vi "BeeperData_Validation.vi"(0 "offset":dbl=131.6, 1 "path":path=path "C:/mtp/Site_Ne_sch/Projects/AVALANCHE/CUSTOM/BeeperData/14251010502229-Beeper_9_50_56.wav", 4 "Upper Cut-Off":dbl=15000.0, 5 "Lower Cut-Off":dbl=2000.0) -> (10 "N Harmonics":i32=1, 12 "Harmonic Array":T1(array[cluster])=[{"detected frequency"=2960.3023758852505, "detected amplitude"=100.09262427578935, "detected phase (deg)"=21.541772749437428}], 13 "error out":errorcluster, 14 "PASS/FAIL 4":bool=TRUE caption="PASS/FAIL", 15 "fundamental frequency":dbl=2934.715709878751 format="%.2p", 16 "fundamental amplitude":dbl=0.025259592284939396, 17 "fundamental dB output":dbl=99.6485267265794, 18 "THD":dbl=9.755635404697069 format="%.2p")   [LabVIEW 2014]
uses:
  <vilib>/express/express analysis/Spectral/Block/exnSpectralBlock spectral measurements peak poly.vi
  <vilib>/express/express analysis/Spectral/Block/exnSpectralBlock spectral measurements peak WFM.vi
  <vilib>/measure/matone.llb/Extract Multiple Tone Information 1 Chan.vi
  <vilib>/measure/matone.llb/Harmonic Distortion Analyzer 1 Chan.vi
  <vilib>/express/express analysis/Spectral/XNode/ExpressSpectralMeasurementsBlockNode.xnode
  <vilib>/measure/NI_MAPro.lvlib
panel:
  out "max index(es)":i32=1
  out "components level":dbl[](array[numeric])=[-2.401233861026392e-07, 0.025259592284939396, 0.002224247422714069, 0.00081423605464637, 0.000593690234948729, 0.00033120473717450035, 5.1228130884612615e-06, 4.283185131983852e-09, 2.0407182090206694e-10] format="%.2p"
  out "Beeper Time Domain AC":waveform(dbl)(graph)={"t0"=timestamp(0.0010416666666666667 s since 1904-01-01), "dt"=2.0833333333333333e-05, "Y"=array[455 elements], "attributes"=variant("NI_ChannelName"=variant(string "Filtered (Extracted)"), "NI_ExpIsRelativeTime"=variant(bool TRUE), "NI_ExpStartTimeStamp"=variant(timestamp timestamp(3493299977.1484375 s since 1904-01-01)), "NI_ExpTimeStamp"=variant(timestamp timestamp(3493299977.1494794 s since 1904-01-01)), "NI_ExpXDimension"=variant(string "t"), "NI_OriginalChannelName"=variant(string "Filtered"))}
  out "FFT Mask":dynamicdata(graph)=[{"t0"=timestamp(-68399 s since 1904-01-01), "dt"=105.49450549450549, "Y"=array[228 elements]}, {"t0"=timestamp(-68399 s since 1904-01-01), "dt"=105.49450549450549, "Y"=[nan, nan, nan, nan, nan, nan, nan, nan, nan, nan, nan, nan, nan, nan, nan, nan, nan, nan, nan, nan, nan, nan, nan, nan, nan, nan, nan, nan, nan, nan, nan, nan, nan, nan, nan, nan, nan, nan, nan, nan, nan, nan, nan, nan, nan, nan, nan, nan, nan, nan, nan, nan, nan, nan, nan, nan, nan, nan, nan, nan, nan, nan, nan, nan, nan, nan, nan, nan, nan, nan, nan, nan, nan, nan, nan, nan, nan, nan, nan, nan, nan, nan, nan, nan, nan, nan, nan, nan, nan, nan, nan, nan, nan, nan, nan, nan, nan, nan, nan, nan, nan, nan, nan, nan, nan, nan, nan, nan, nan, nan, nan, nan, nan, nan, nan, nan, nan, nan, nan, nan, nan, nan, nan, nan, nan, nan, nan, nan, nan, nan, nan, nan, nan, nan, nan, nan, nan, nan, nan, nan, nan, nan, nan, nan, nan, nan, nan, nan, nan, nan, nan, nan, nan, nan, nan, nan, nan, nan, nan, nan, nan, nan, nan, nan, nan, nan, nan, nan, nan, nan, nan, nan, nan, nan, nan, nan, nan, nan, nan, nan, nan, nan, nan, nan, nan, nan, nan, nan, nan, nan, nan, nan, nan, nan, nan, nan, nan, nan, nan, nan, nan, nan, nan, nan, nan, nan, nan, nan, nan, nan, nan, nan, nan, nan, nan, nan, nan, nan, nan, nan, nan, nan, nan, nan, nan, nan, nan, nan], "attributes"=variant("NI_ChannelName"=variant(string "Failures"))}, {"t0"=timestamp(-68399 s since 1904-01-01), "dt"=105.49450549450549, "Y"=[3.0, 3.0, 3.0, 3.0, 3.0, 2.9700353311878396, 2.916806756284134, 2.8635781813804284, 2.8103496064767235, 2.7571210315730177, 2.7038924566693128, 2.650663881765607, 2.5974353068619016, 2.5442067319581962, 2.490978157054491, 2.4377495821507855, 2.38452100724708, 2.331292432343375, 2.2780638574396694, 2.224835282535964, 2.1716067076322587, 2.118378132728553, 2.065149557824848, 2.011920982921142, 70.0, 70.0, 70.0, 70.0, 70.0, 70.0, 70.0, 70.0, 70.0, 70.0, 2.0, 2.0, 2.0, 2.0, 2.0, 2.0, 2.0, 2.0, 2.0, 2.0, 2.0, 2.0, 2.0, 2.0, 2.0, 2.0, 2.0, 2.0, 36.285714285714114, 50.0, 50.0, 50.0, 50.0, 50.0, 50.0, 50.0, 50.0, 50.0, 10.967032967033415, 2.0, 2.0, 2.0, 2.0, 2.0, 2.0, 2.0, 2.0, 2.0, 2.0, 2.0, 2.0, 2.0, 2.0, 2.0, 2.0, 2.0, 2.0, 20.0, 20.0, 20.0, 20.0, 20.0, 20.0, 20.0, 20.0, 20.0, 20.0, 2.0, 2.0, 2.0, 2.0, 2.0, 2.0, 2.0, 2.0, 2.0, 2.0, 2.0, 2.0, 2.0, 2.0, 2.0, 2.0, 2.0, 2.0, 2.0, 2.0, 2.0, 2.0, 2.0, 2.0, 2.0, 2.0, 2.0, 2.0, 2.0, 2.0, 2.0, 2.0, 2.0, 2.0, 2.0, 2.0, 2.0, 2.0, 2.0, 2.0, 2.0, 2.0, 2.0, 2.0, 2.0, 2.0, 2.0, 2.0, 2.0, 2.0, 2.0, 2.0, 2.0, 2.0, 2.0, 2.0, 2.0, 2.0, 2.0, 2.0, 2.0, 2.0, 2.0, 2.0, 2.0, 2.0, 2.0, 2.0, 2.0, 2.0, 2.0, 2.0, 2.0, 2.0, 2.0, 2.0, 2.0, 2.0, 2.0, 2.0, 2.0, 2.0, 2.0, 2.0, 2.0, 2.0, 2.0, 2.0, 2.0, 2.0, 2.0, 2.0, 2.0, 2.0, 2.0, 2.0, 2.0, 2.0, 2.0, 2.0, 2.0, 2.0, 2.0, 2.0, 2.0, 2.0, 2.0, 2.0, 2.0, 2.0, 2.0, 2.0, 2.0, 2.0, 2.0, 2.0, 2.0, 2.0, 2.0, 2.0, 2.0, 2.0, 2.0, 2.0, 2.0, 2.0, 2.0, 2.0, 2.0, 2.0, 2.0, 2.0, 2.0, 2.0, 2.0, 2.0, 2.0], "attributes"=variant("NI_ChannelName"=variant(string "Upper Limit"))}, {"t0"=timestamp(-68399 s since 1904-01-01), "dt"=105.49450549450549, "Y"=[0.0, 0.0, 0.0, 0.0, 0.0, 0.0, 0.0, 0.0, 0.0, 0.0, 0.0, 0.0, 0.0, 0.0, 0.0, 0.0, 0.0, 0.0, 0.0, 0.0, 0.0, 0.0, 0.0, 0.0, 0.0, 0.0, 0.0, 0.0, 0.0, 0.0, 0.0, 0.0, 0.0, 0.0, 0.0, 0.0, 0.0, 0.0, 0.0, 0.0, 0.0, 0.0, 0.0, 0.0, 0.0, 0.0, 0.0, 0.0, 0.0, 0.0, 0.0, 0.0, 0.0, 0.0, 0.0, 0.0, 0.0, 0.0, 0.0, 0.0, 0.0, 0.0, 0.0, 0.0, 0.0, 0.0, 0.0, 0.0, 0.0, 0.0, 0.0, 0.0, 0.0, 0.0, 0.0, 0.0, 0.0, 0.0, 0.0, 0.0, 0.0, 0.0, 0.0, 0.0, 0.0, 0.0, 0.0, 0.0, 0.0, 0.0, 0.0, 0.0, 0.0, 0.0, 0.0, 0.0, 0.0, 0.0, 0.0, 0.0, 0.0, 0.0, 0.0, 0.0, 0.0, 0.0, 0.0, 0.0, 0.0, 0.0, 0.0, 0.0, 0.0, 0.0, 0.0, 0.0, 0.0, 0.0, 0.0, 0.0, 0.0, 0.0, 0.0, 0.0, 0.0, 0.0, 0.0, 0.0, 0.0, 0.0, 0.0, 0.0, 0.0, 0.0, 0.0, 0.0, 0.0, 0.0, 0.0, 0.0, 0.0, 0.0, 0.0, 0.0, 0.0, 0.0, 0.0, 0.0, 0.0, 0.0, 0.0, 0.0, 0.0, 0.0, 0.0, 0.0, 0.0, 0.0, 0.0, 0.0, 0.0, 0.0, 0.0, 0.0, 0.0, 0.0, 0.0, 0.0, 0.0, 0.0, 0.0, 0.0, 0.0, 0.0, 0.0, 0.0, 0.0, 0.0, 0.0, 0.0, 0.0, 0.0, 0.0, 0.0, 0.0, 0.0, 0.0, 0.0, 0.0, 0.0, 0.0, 0.0, 0.0, 0.0, 0.0, 0.0, 0.0, 0.0, 0.0, 0.0, 0.0, 0.0, 0.0, 0.0, 0.0, 0.0, 0.0, 0.0, 0.0, 0.0, 0.0, 0.0, 0.0, 0.0, 0.0, 0.0, 0.0, 0.0, 0.0, 0.0, 0.0, 0.0, 0.0, 0.0, 0.0, 0.0, 0.0, 0.0], "attributes"=variant("NI_ChannelName"=variant(string "Lower Limit"))}]
  out "Beeper Time Domain DC":waveform(dbl)(graph)={"t0"=timestamp(0 s since 1904-01-01), "dt"=2.0833333333333333e-05, "Y"=array[505 elements]}
  out "FFT Peak":cluster{"f0":dbl, "df":dbl, "magnitude":dbl[]}(graph)={"f0"=0.0, "df"=105.49450549450549, "magnitude"=[1.6018368008824488e-07, 2.739165277402443e-07, 3.985203981044255e-07, 5.917708316720877e-07, 8.748145112128303e-07, 1.3010814410825855e-06, 2.0802062107375216e-06, 2.790134744566662e-06, 5.753123783912797e-06, 1.4763146182645159e-05, 4.238164606283932e-06, 0.00012007636572453463, 0.00045236073044393853, 0.002934004193699415, 0.00618501386299634, 0.0064880498159982855, 0.004538550933487086, 0.005199055511354578, 0.006129575152514394, 0.006903653173956658, 0.00730576670286189, 0.007351995343235854, 0.007013327451583518, 0.006509554866980719, 0.006228470853974282, 0.0059152113548739315, 0.005498597813254141, 0.016062761736819666, 0.02472840707265435, 0.014786365312579881, 0.00239181992405032, 0.0021946637725328354, 0.0016716329640382012, 0.0022855801600055793, 0.0020901873459184686, 0.0017113901006194504, 0.001620746494749405, 0.0015562218927555732, 0.0013615690730541976, 0.0012180416934189037, 0.001119963237415986, 0.0012235355092325316, 0.004180665312898901, 0.0043012327175093144, 0.001612474254557478, 0.0014550970818332164, 0.002184396771928845, 0.0015683282438508053, 0.0015113981640458374, 0.0018553299437078332, 0.001432021634658514, 0.0012923059165754112, 0.0011823857826419426, 0.0010576757189758696, 0.0011219595762485385, 0.0004573132325211268, 0.0015561090460205571, 0.0021222291843564127, 0.0013223324797204017, 0.0011297547810841938, 0.0009469486200130573, 0.001072221032431467, 0.0010140248379210456, 0.0009535198860453821, 0.0009713855535785712, 0.0009733887927467716, 0.0009231871530565895, 0.0008862720858397985, 0.0008697663729143937, 0.0008808024231401676, 0.0008311296857765208, 0.0007683276179268573, 0.0007961849804113151, 0.0007876581727953233, 0.0007888359132087923, 0.000769776362911128, 0.0007402871142191691, 0.0007523865145557025, 0.0007307766379216526, 0.0007212053921743106, 0.0007221095514331676, 0.0007113072058043807, 0.0007071121006542068, 0.0006742963491071851, 0.0006427924843893649, 0.0006870497263242136, 0.0006749536371613217, 0.0006613102492586514, 0.0006489994908067029, 0.0006293390742419889, 0.0006363895989919498, 0.0006288592489611338, 0.0006141636133007902, 0.0005998170467609775, 0.000606898767172136, 0.0006100954906706817, 0.0005950655468311286, 0.0005687631384143958, 0.000645402197941972, 0.0006093938618635512, 0.0005440439587081989, 0.0005491501408034803, 0.0005471993333521795, 0.000555731215915673, 0.0005448049609387473, 0.0005268014591564282, 0.0005276165035064028, 0.0005193301431807729, 0.0005176891895592861, 0.0005071285001398295, 0.0005128221736897446, 0.0004946929370202132, 0.00020655127828846196, 0.0005833042883385348, 0.0005986223100015384, 0.000514062759255501, 0.0005162656836314005, 0.0004947426900875093, 0.0004900740942022137, 0.0005128959777501746, 0.0004962426346107286, 0.0004480936091845419, 0.0004677545173529926, 0.0004916103843928828, 0.00046833095017899206, 0.0004561521011779545, 0.0005351975121194499, 0.00048074459952987807, 0.0004019354125465926, 0.0004328421538882473, 0.0004177256245699992, 0.000401433108737401, 0.00040727619876232895, 0.00039014492249631315, 0.00037122537926854093, 0.0003572568717356956, 0.0003347011841836008, 0.000317645831002189, 0.00029499272337436887, 0.0002655709639012852, 0.0002456444610692289, 0.0002979351613877896, 0.0002488337977494649, 0.00021442893771735202, 0.00019253195485906686, 0.00016871746475827094, 0.00014708573773234747, 0.0001316727205698442, 0.00011475346989928615, 9.999567957957976e-05, 8.355183515284517e-05, 7.455418882715166e-05, 6.299284392853712e-05, 5.120665746323067e-05, 4.774908197114614e-05, 4.391330974930402e-05, 3.181851168252048e-05, 2.7269674200429926e-05, 2.221941603966412e-05, 1.8772239623046817e-05, 1.525105733418944e-05, 1.268089996340142e-05, 1.0235236333480283e-05, 8.551419418824312e-06, 6.9648649934696785e-06, 5.701748469266331e-06, 4.6962748957860825e-06, 3.922975065968365e-06, 3.067600106921259e-06, 2.530168944911267e-06, 2.068764944567118e-06, 1.666524485415195e-06, 1.3596624429221118e-06, 1.0836402074972496e-06, 8.989168769003971e-07, 7.197165570656004e-07, 5.481961280152284e-07, 4.472978961163214e-07, 3.637035768405892e-07, 2.787960899093122e-07, 2.1910979507048683e-07, 1.7296865493676617e-07, 1.3617842183839526e-07, 1.0468236401971942e-07, 8.287618712431156e-08, 6.33389189173673e-08, 4.785647426903807e-08, 3.652941249268399e-08, 3.04849648281208e-08, 2.265482254064642e-08, 1.6678952098245288e-08, 1.1962707544068855e-08, 9.019654193848143e-09, 7.257736329668531e-09, 4.61540575313361e-09, 3.0634685329644013e-09, 3.0153156852308272e-09, 1.981309720589669e-09, 7.567519387012121e-10, 1.1198464971128534e-09, 1.0079345420920498e-09, 8.701582864538078e-10, 1.3927584173258147e-09, 1.0723596774364627e-09, 3.4216758540295366e-10, 4.429352546738541e-10, 4.4336447100413793e-10, 3.6791998346199263e-10, 3.684405363850955e-10, 3.7838754731252655e-10, 3.5788638668105033e-10, 3.4703595026039633e-10, 3.4356000066506645e-10, 3.3494943254810104e-10, 3.269648763852098e-10, 3.208964950838077e-10, 3.147313728415835e-10, 3.0891418933647756e-10, 3.0373615893461565e-10, 2.9901971109520886e-10, 2.9478708873471836e-10, 2.9106814410454076e-10, 2.878628402777732e-10, 2.851786402689724e-10, 2.8302272856028055e-10, 2.814006053361294e-10, 2.803166559304008e-10, 2.797739135846308e-10]}
  # "Trigger at 0.8"
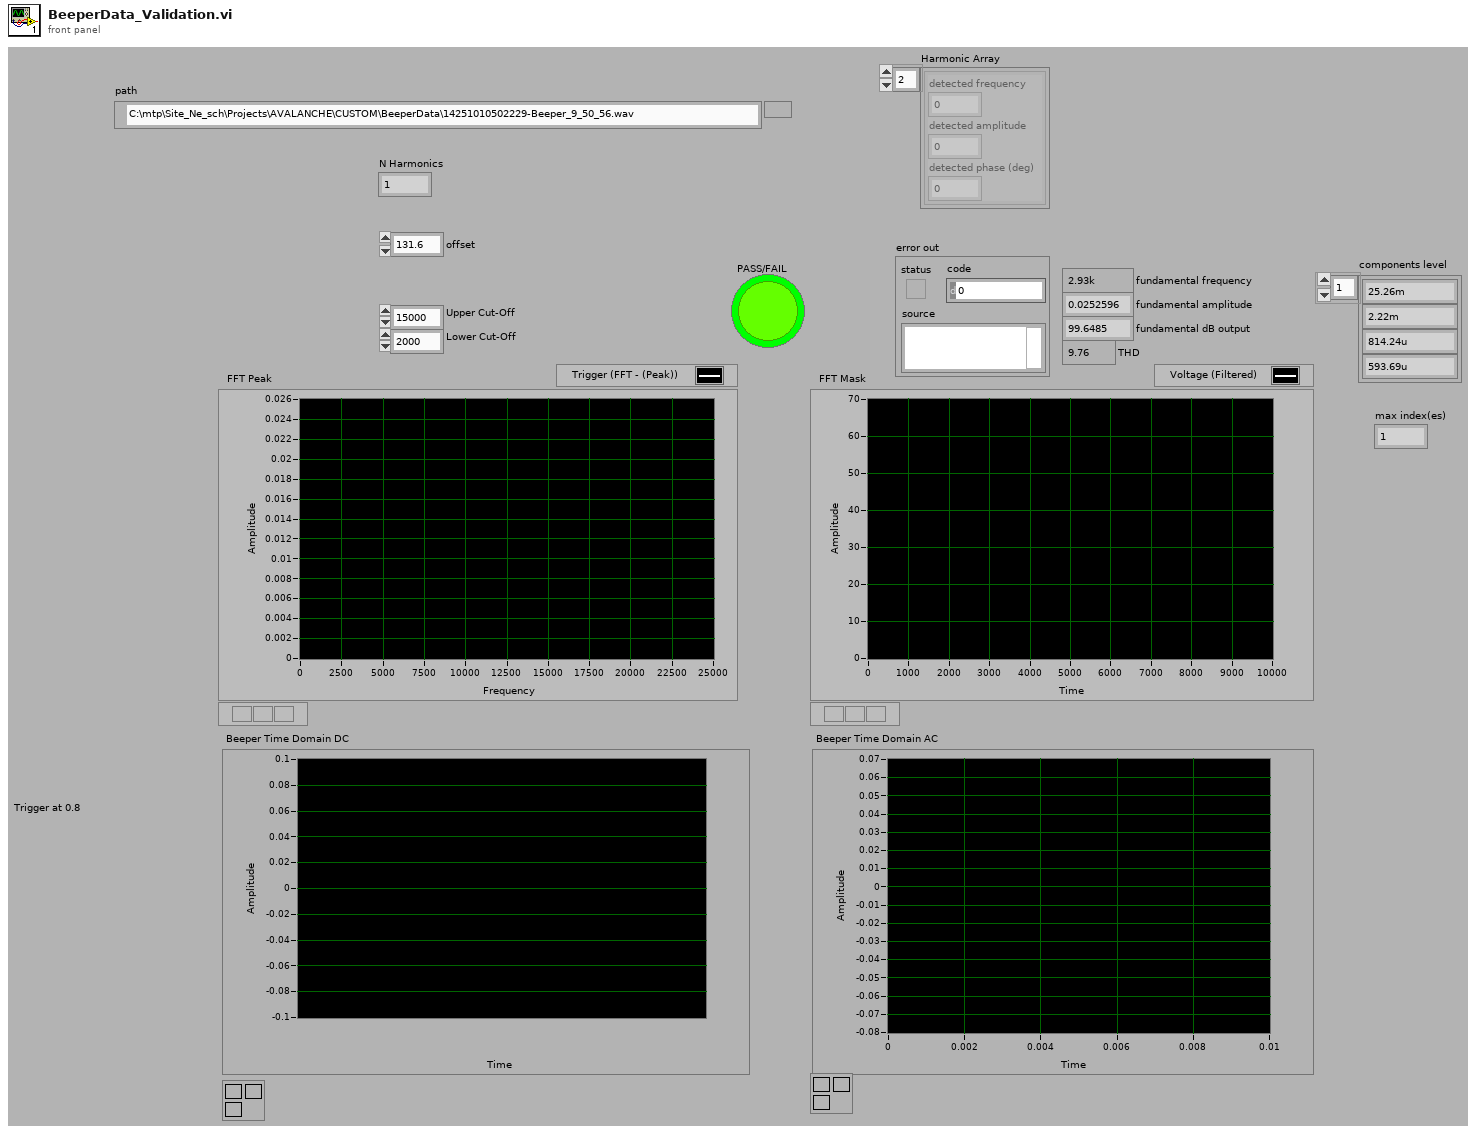
[diagram p1: front panel]
types:
  T1 = cluster{"detected frequency":dbl, "detected amplitude":dbl, "detected phase (deg)":dbl}[]
  T2 = cluster{"averaging mode":u16, "weighting mode":u16, "number of averages":u32}
  T3 = cluster{"dB On (F)":bool, "unwrap phase (F)":bool, "convert to degree (F)":bool}
  T4 = cluster{"approx freq. (optional)":dbl, "search (+/- % of Fsampl.)":dbl}
  T5 = enum32{"none", "input signal", "detected signal", "residual signal"}
  T6 = enum16{"none", "input signal", "fundamental signal", "residual signal", "harmonics only", "noise and spurs"}
  T7 = cluster{"detected frequency":dbl, "detected amplitude":dbl, "detected phase (deg)":dbl}
  T8 = cluster{"detected frequency":dbl, dbl, "detected phase (deg)":dbl}
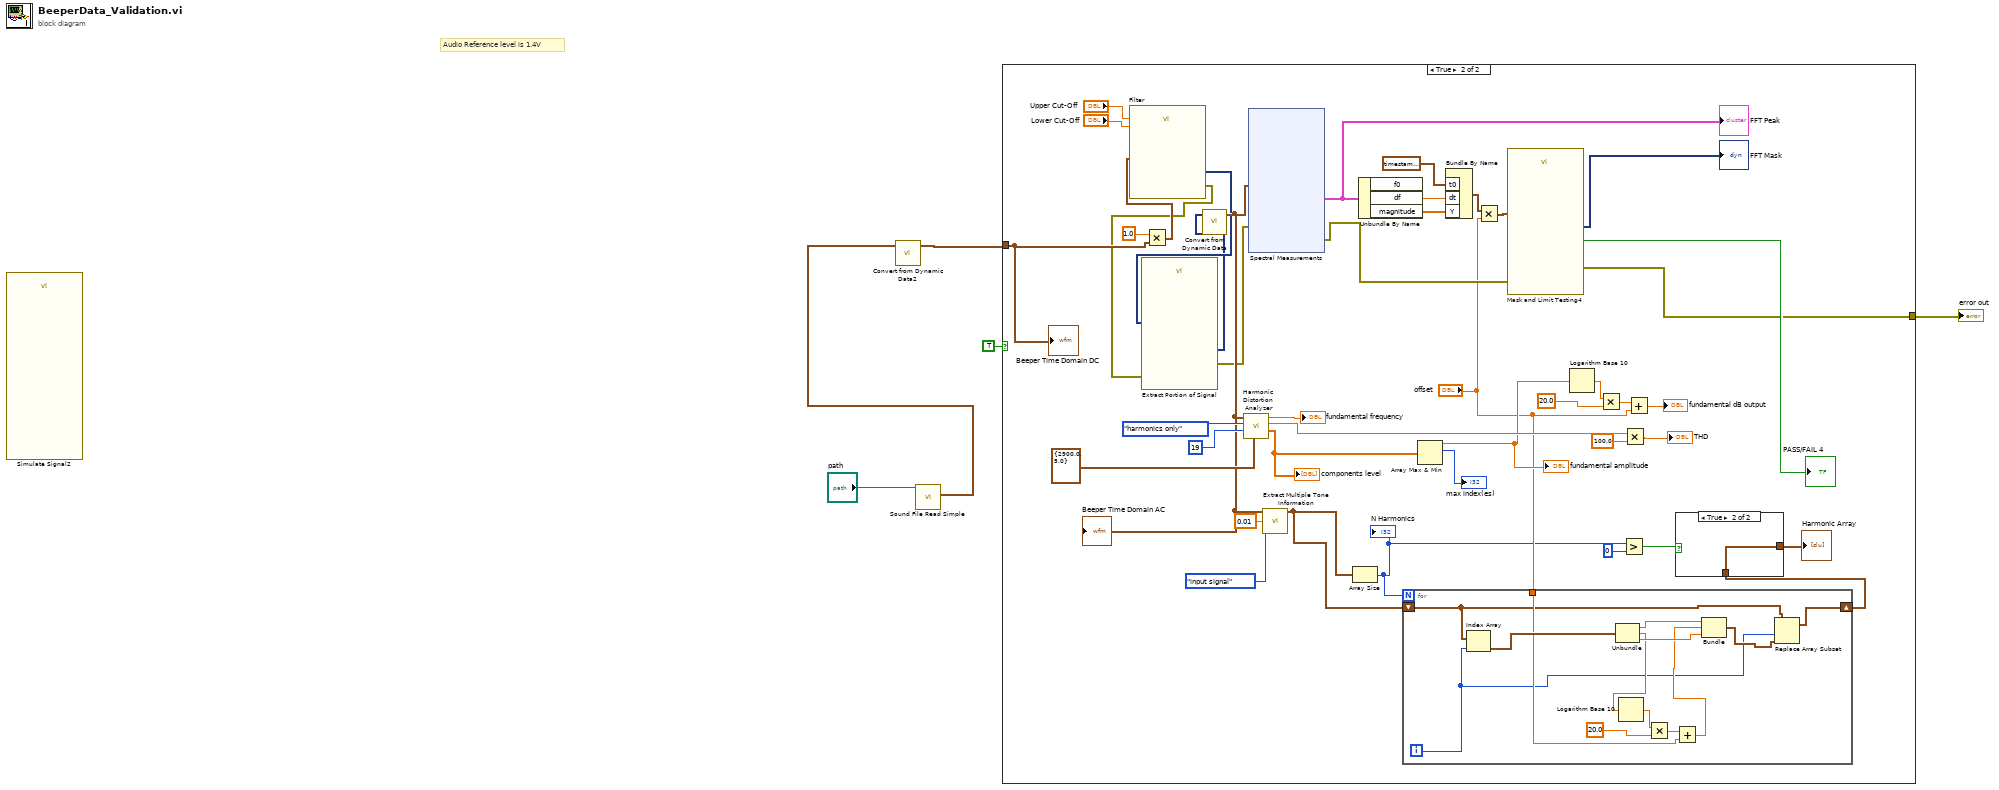
[diagram p0: block diagram]
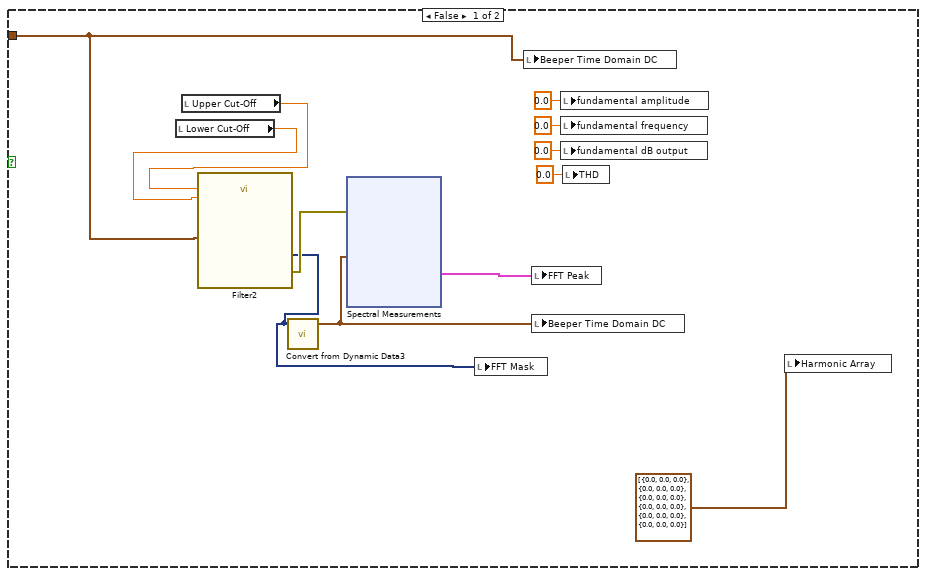
[diagram p2: hidden frame]
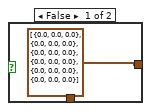
[diagram p3: hidden frame]
diagram:
  # "Audio Reference level is 1.4V"
  n1 = call "Simulate Signal2"() -> ()  [unwired: 14 in, 2 out]
  n2 = call <vilib>:"Sound File Read Simple.vi"("path"="path") -> ("data"=w2:waveform(dbl)[])  [unwired: 7 in, 3 out]
  n3 = call "Convert from Dynamic Data2"("Dynamic Data Type"=w2) -> ("Waveform"=w3:waveform(dbl))  [unwired: 3 in]
  n4 = case shown="True" TRUE {
    tunnel: w3 -> [w11 w47]
    tunnel: [_ w68] -> w5
    frame False {
      n5 = local read "Lower Cut-Off"() -> (w8:dbl)
      n6 = local read "Upper Cut-Off"() -> (w7:dbl)
      n7 = call "Filter2"("Lower Cut-Off"=w8, "Upper Cut-Off"=w7, "Signal"=w11) -> ("error out"=w12:errorcluster, "Filtered Signal"=w9:dynamicdata)  [unwired: 7 in]
      n8 = call "Convert from Dynamic Data3"("Dynamic Data Type"=w9) -> ("Waveform"=w6:waveform(dbl))  [unwired: 3 in]
      n9 = xnode "Spectral Measurements"("Signals"=w6, "error in (no error)"=w12) -> ("FFT - (Peak)"=w10:cluster{"f0":dbl, "df":dbl, "magnitude":dbl[]})  [unwired: 2 out]
      n10 = local write "FFT Mask"(w9) -> ()
      n11 = local write "Beeper Time Domain DC"(w11) -> ()
      n12 = local write "FFT Peak"(w10) -> ()
      n13 = local write "Beeper Time Domain DC"(w6) -> ()
      n14 = local write "fundamental amplitude"(0.0 ("fundamental amplitude")) -> ()
      n15 = local write "fundamental frequency"(0.0 ("fundamental frequency")) -> ()
      n16 = local write "fundamental dB output"(0.0 ("fundamental dB output")) -> ()
      n17 = local write "THD"(0.0 ("THD")) -> ()
      n18 = local write "Harmonic Array"(T1 [{"detected frequency"=0.0, "detected amplitude"=0.0, "detected phase (deg)"=0.0}, {"detected frequency"=0.0, "detected amplitude"=0.0, "detected phase (deg)"=0.0}, {"detected frequency"=0.0, "detected amplitude"=0.0, "detected phase (deg)"=0.0}, {"detected frequency"=0.0, "detected amplitude"=0.0, "detected phase (deg)"=0.0}, {"detected frequency"=0.0, "detected amplitude"=0.0, "detected phase (deg)"=0.0}, {"detected frequency"=0.0, "detected amplitude"=0.0, "detected phase (deg)"=0.0}] ("multiple tone information")) -> ()
    }
    frame True {
      n19 = Multiply(x=1.0, y=w47) -> (x*y=w48:waveform(dbl))
      n20 = call "Filter"("Lower Cut-Off"="Lower Cut-Off", "Upper Cut-Off"="Upper Cut-Off", "Signal"=w48) -> ("error out"=w28:errorcluster, "Filtered Signal"=w31:dynamicdata)  [unwired: 7 in]
      n21 = call "Extract Portion of Signal"("error in (no error)"=w28, "Signals"=w31) -> ("error out"=w29:errorcluster, "Section"=w30:dynamicdata)  [unwired: 8 in]
      n22 = call "Convert from Dynamic Data"("Dynamic Data Type"=w30) -> ("Waveform"=w41:waveform(dbl))  [unwired: 3 in]
      "Beeper Time Domain AC" <- w41
      n23 = call-poly <vilib>:"Harmonic Distortion Analyzer.vi"("advanced search"=T4 {"approx freq. (optional)"=2900.0, "search (+/- % of Fsampl.)"=5.0}, "highest harmonic"=19, "export mode"=T6."harmonics only" ("export signals"), "signal in"=w41) -> ("components level"=w45:dbl[], "THD"=w53:dbl, "detected fundamental frequency"=→"fundamental frequency":dbl)  [unwired: 2 in, 3 out]
      "components level" <- w45
      n24 = xnode "Spectral Measurements"("Signals"=w41, "error in (no error)"=w29) -> ("FFT - (Peak)"=w42:cluster{"f0":dbl, "df":dbl, "magnitude":dbl[]}, "error out"=w49:errorcluster)  [unwired: 1 out]
      "FFT Peak" <- w42
      n25 = call-poly <vilib>:"Extract Multiple Tone Information.vi"("time signal in"=w41, "export mode"=T5."input signal", "threshold"=0.01) -> ("multiple tone information"=w38:T1)  [unwired: 10 in, 2 out]
      n26 = Array Size(array=w38) -> (size(s)=w36:i32)
      "N Harmonics" <- w36
      n27 = Unbundle By Name(w42) -> ("df"=w66:dbl, "magnitude"=w65:dbl[])  [unwired: 1 out]
      n28 = for {
        N: w36 -> [_]
        tunnel: "offset" -> [w76]
        shift-right: [w74] -> w33
        shift-left: w38 -> [w73]
        i -> [w75]
        n29 = Index Array(array=w73, index=w75) -> (element=w85:T7)
        n30 = Unbundle(w85) -> ("detected frequency"=w84:dbl, "detected amplitude"=w78:dbl, "detected phase (deg)"=w83:dbl)
        n31 = Logarithm Base 10(1:w78) -> (0:w81:dbl)
        n32 = Multiply(x=w81, y=20.0) -> (x*y=w79:dbl)
        n33 = Add(x=w79, y=w76) -> (x+y=w77:dbl)
        n34 = Bundle("detected frequency"=w84, w77, "detected phase (deg)"=w83) -> (w82:T8)  [unwired: 1 in]
        n35 = Replace Array Subset(array=w73, new element=w82, index=w75) -> (w74:T1)
      }
      n36 = Array Max & Min(array=w45) -> (max value=w52:dbl, max index (indices)=→"max index(es)":i32)  [unwired: 2 out]
      "fundamental amplitude" <- w52
      n37 = Bundle By Name("t0"=timestamp(-68399 s since 1904-01-01), "dt"=w66, "Y"=w65) -> (w50:waveform(dbl))  [unwired: 1 in]
      n38 = Multiply(x=w50, y="offset") -> (x*y=w51:waveform(dbl))
      n39 = call "Mask and Limit Testing4"("error in"=w49, "Signals"=w51) -> ("error out"=w68:errorcluster, "Passed"=→"PASS/FAIL 4":bool, "Tested Signals"=→"FFT Mask":dynamicdata)  [unwired: 6 in, 1 out]
      n40 = Logarithm Base 10(1:w52) -> (0:w62:dbl)
      n41 = Multiply(x=w62, y=20.0) -> (x*y=w60:dbl)
      n42 = Greater?(x=w36, y=0) -> (0:w34:bool)
      n43 = Multiply(x=w53, y=100.0) -> (x*y=→"THD":dbl)
      n44 = Add(x=w60, y="offset") -> (x+y=→"fundamental dB output":dbl)
      n45 = case shown="True" w34 {
        tunnel: w33 -> [_ w72]
        tunnel: [T1 [{"detected frequency"=0.0, "detected amplitude"=0.0, "detected phase (deg)"=0.0}, {"detected frequency"=0.0, "detected amplitude"=0.0, "detected phase (deg)"=0.0}, {"detected frequency"=0.0, "detected amplitude"=0.0, "detected phase (deg)"=0.0}, {"detected frequency"=0.0, "detected amplitude"=0.0, "detected phase (deg)"=0.0}, {"detected frequency"=0.0, "detected amplitude"=0.0, "detected phase (deg)"=0.0}, {"detected frequency"=0.0, "detected amplitude"=0.0, "detected phase (deg)"=0.0}] ("multiple tone information") w72] -> w32
        frame False {
        }
        frame True {
        }
      }
      "Harmonic Array" <- w32
      "Beeper Time Domain DC" <- w47
    }
  }
  "error out" <- w5
